vi "List Reserved IDs.vi"(8 "error in (no error)":errorcluster, 11 "Client in":refnum<class "Client.lvclass">) -> (0 "error out":errorcluster, 2 "Reserved PacketIDs":u16[](array[numeric]) format="%016b", 3 "Client out":refnum<class "Client.lvclass">)   [LabVIEW 2013, in "MQTT Server.lvlib" / "Client.lvclass"]
uses:
  Client.lvclass
  Client.lvclass/Client.ctl
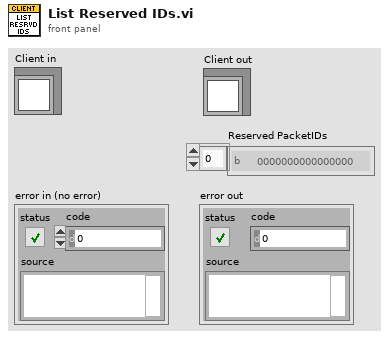
[diagram p1: front panel]
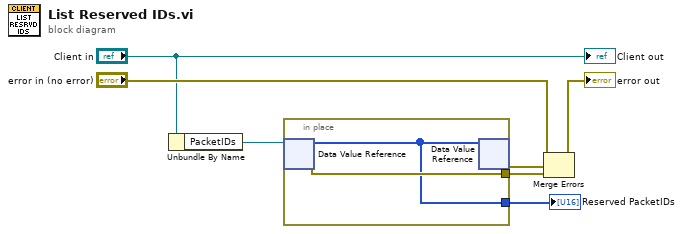
[diagram p0: block diagram]
diagram:
  n1 = Unbundle By Name("Client in") -> ("PacketIDs"=w3:refnum<data-value>)
  n2 = in-place {
    in-place-border: [w9] -> w4
    in-place-border: [w8] -> w1
    n3 = in-place-dvr #1(w3) -> (w8:u16[], w9:errorcluster)
    n4 = in-place-dvr #1(w8) -> (w5:errorcluster)  [unwired: 1 out]
  }
  "Reserved PacketIDs" <- w1
  n5 = Merge Errors("error in (no error)", w5, w4) -> (→"error out":errorcluster)
  "Client out" <- "Client in"
